vi "Pcre2JitStackCreate.vi"(8 "error in":errorcluster, 10 "MaxSize (1 MiB)":u64=1048576, 11 "StartSize (32 KiB)":u64=32768) -> (0 "error out":errorcluster, 3 "pJitStack":u64 format="%.0x")   [LabVIEW 2021, in "libpcre2-8.lvlib"]
uses:
  libpcre2-8.lvlib
  libpcre2-8-x32.dll
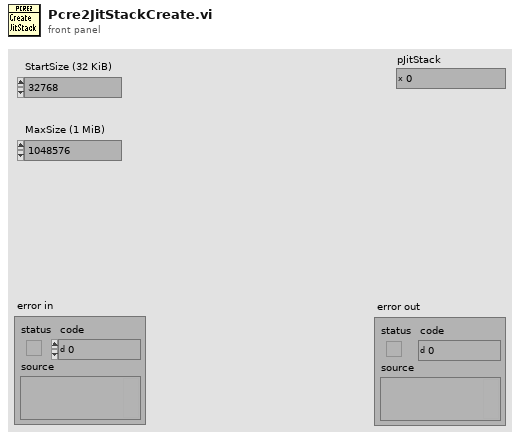
[diagram p1: front panel]
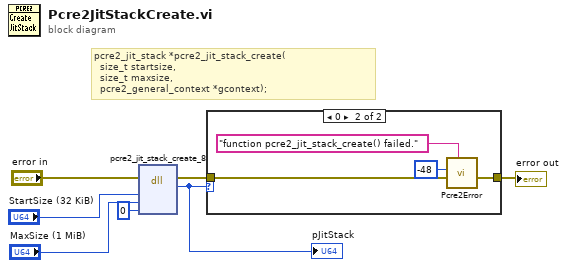
[diagram p0: block diagram]
diagram:
  # "pcre2_jit_stack *pcre2_jit_stack_create(\n  size_t startsize,\n  size_t maxsize,\n  pcre2_general_context *gcontext);"
  n1 = dll-call lib="libpcre2-8-x*.dll" fn="pcre2_jit_stack_create_8"(error in="error in", "startsize"="StartSize (32 KiB)", "maxsize"="MaxSize (1 MiB)", "gcontext"=u64 0) -> (error out=w3:errorcluster, "JitStack"=w2:u64)  [unwired: 5 in, 1 out]
  "pJitStack" <- w2
  n2 = case shown="0" w2 {
    tunnel: w3 -> [w8 w11]
    tunnel: [w8 w10] -> w1
    frame Default {
    }
    frame 0 {
      n3 = call "Pcre2Error.vi"("message"="function pcre2_jit_stack_create() failed.", "error in"=w11, "ErrorCode"=-48) -> ("error out"=w10:errorcluster)  [unwired: 8 in]
    }
  }
  "error out" <- w1
